vi "Send Divide.vi"(7 "Message Priority":T1=enum."Normal", 8 "error in (no error)":errorcluster, 11 "Actor Framework.lvlib:Send Queue":refnum<class "Message Enqueuer.lvclass">) -> (0 "error out":errorcluster)   [LabVIEW 2012, in "Divide Msg.lvclass"]
uses:
  Divide Msg.lvclass
  <vilib>/ActorFramework/Message Enqueuer/Message Priority.ctl
  <vilib>/ActorFramework/Message Enqueuer/Message Enqueuer.lvclass
  <vilib>/ActorFramework/Message Enqueuer/Message Enqueuer.lvclass/Message Enqueuer.ctl
  <vilib>/ActorFramework/Message Priority Queue/Priority Enqueue.vi
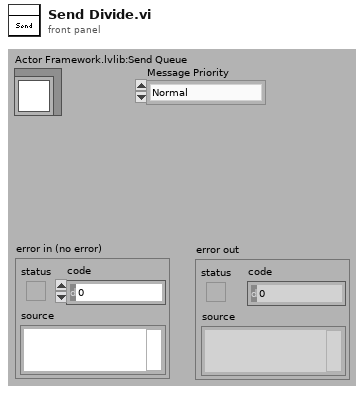
[diagram p1: front panel]
types:
  T1 = typedef "Actor Framework.lvlib/Message Enqueuer.lvclass/Message Priority.ctl" = enum16{"Low", "Normal", "High"}
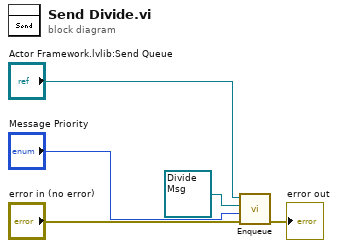
[diagram p0: block diagram]
diagram:
  n1 = call <vilib>:"Enqueue.vi"("error in (no error)"="error in (no error)", "Message Priority (Normal)"="Message Priority", "Message"=refnum<class "Divide Msg.lvclass"> refnum ("Object"), "Message Enqueuer in"="Actor Framework.lvlib:Send Queue") -> ("error out"=→"error out":errorcluster)  [unwired: 6 in, 1 out]
